vi "Call Serial Decoder.vi"(0 "Write Value":string="108500", 1 "wait ms":u32=500, 2 "VISA resource name":refnum<visa-resource-name>, 3 "error in":errorcluster={"status"=FALSE, "code"=-1073807343, "source"=""}) -> (4 "Data Not Good":bool, 5 "Data Read":T1={"Date"="03/29/13", "Time"="14:47:22", "CO2- ppm"=753, "Last Ctrl Word"=5276928, "O2-1 ppm"=209104, "O2-2 ppm"=209104, "Temp MB"=20.41, "Temp Sensor Modulr"=21.85, "Press mB"=835.52} {"Last Ctrl Word" format="%.0x"}, 6 "VISA resource name out":refnum<visa-resource-name>, 7 "error out":errorcluster={"status"=FALSE, "code"=-1073807343, "source"=""})   [LabVIEW 2013]
panel:
  out "read buffer":string="03/29/13,14:47:22,753, 00508500, 209104, 209104, 20.41, 21.85, 835.52\r\n"
  out "concatenated string":string="W108500\rR"
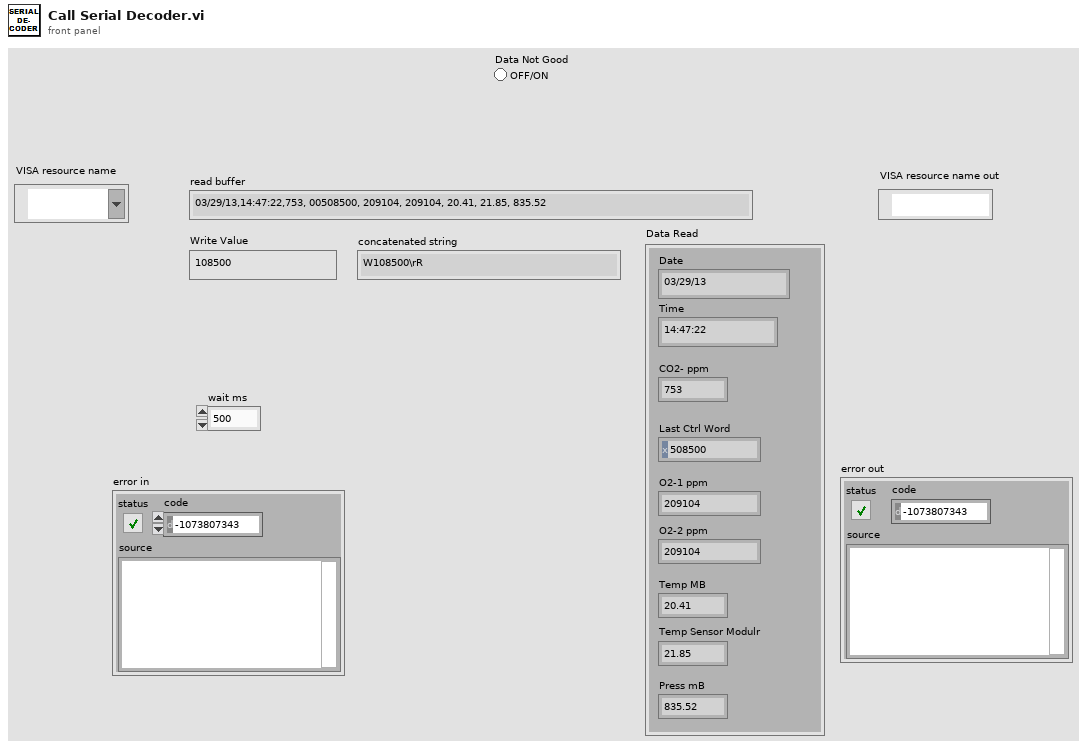
[diagram p1: front panel]
types:
  T1 = cluster{"Date":string, "Time":string, "CO2- ppm":u32, "Last Ctrl Word":u32, "O2-1 ppm":u32, "O2-2 ppm":u32, "Temp MB":sgl, "Temp Sensor Modulr":sgl, "Press mB":sgl}
  T2 = cluster{"default value 1":string, "default value 1":string, "default value 5":u32, "default value 5":u32, "default value 5":u32, "default value 5":u32, "default value 7":sgl, "default value 7":sgl, "default value 7":sgl}
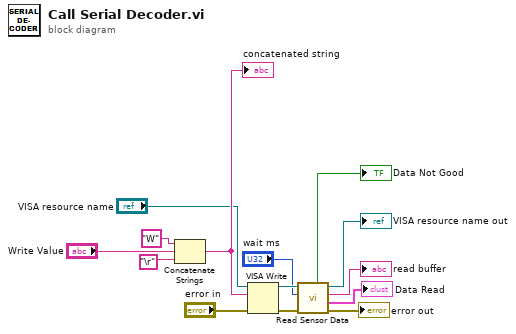
[diagram p0: block diagram]
diagram:
  n1 = Concatenate Strings("W" ("string"), "Write Value", "\r") -> (w14:string)
  "concatenated string" <- w14
  n2 = VISA Write(VISA resource name="VISA resource name", write buffer=w14, error in (no error)="error in") -> (VISA resource name out=w4:refnum<visa-resource-name>, error out=w3:errorcluster)  [unwired: 1 out]
  n3 = call "Read Sensor Data.vi"("error in (no error)"=w3, "wait ms"="wait ms", "VISA Refnum in"=w4) -> ("error out"=→"error out":errorcluster, "DataOut"=→"Data Read":T2, "read buffer"=→"read buffer":string, "VISA Refnum out"=→"VISA resource name out":refnum<visa-resource-name>, "Data Not Good"=→"Data Not Good":bool)  [unwired: 4 in]
